vi "GA_Calculate Fitnesses.vi"(6 "Parameters":T1={"Population size"=100, "Generations no."=500, "Significant digits"=4, "Crossover probabality"=0.85, "Mutation mode"=enum."one-point, fixed rate", "Use Gray code?"=FALSE, "Mutation rate"=0.05, "Min mutation rate"=0.0005, "Max mutation rate"=0.25, "Reproduction plan"=enum."Steady-state-replace-worst", "Elitism"=FALSE, "Fmax"=1} {"Max mutation rate" min=0.0 max=1.0; "Min mutation rate" min=0.0 max=1.0; "Mutation rate" min=0.0 max=1.0; "Crossover probabality" min=0.0 max=1.0; "Significant digits" min=1; "Generations no." min=1; "Population size" min=1}, 7 "Fitness Function":T3, 11 "Population in":T2) -> (3 "Population out":T2)   [LabVIEW 2016, in "Optimal Frequency Bands Search.lvlib" / "GeneticAlgorithm.lvlib"]
doc: "Рассчитать значения функции приспособленности"
uses:
  GeneticAlgorithm.lvlib
  GA_tFitness Function.ctl
  GA_tPopulation.ctl
  GA_tParameters.ctl
  particle_swarm_opt/ParticleSwarm.lvlib
panel:
  # "This VI is a part of BCI Design library, http://www.ru-bci.org \nCopyright © 2020, Sotnikov Peter, All rights reserved. License: GNU GPLv3"
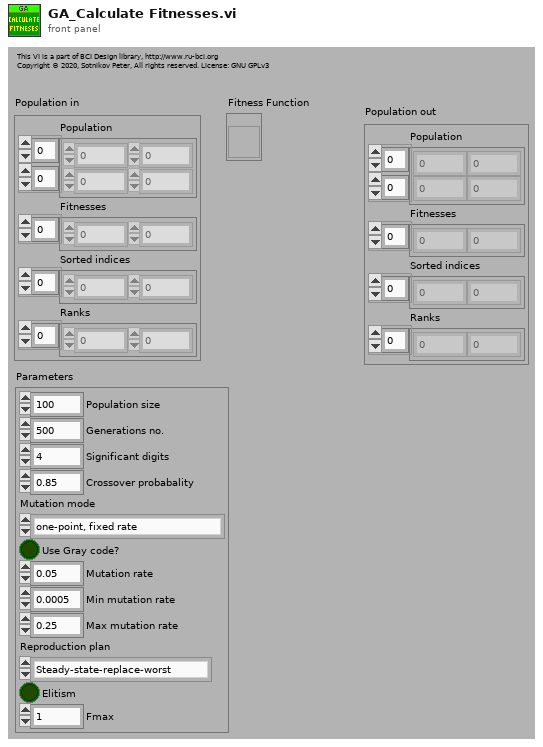
[diagram p1: front panel]
types:
  T1 = typedef "Optimal Frequency Bands Search.lvlib/GeneticAlgorithm.lvlib/GA_tParameters.ctl" = cluster{"Population size":i32, "Generations no.":i32, "Significant digits":i32, "Crossover probabality":dbl, "Mutation mode":enum16{"one-point, fixed rate", "one-point, fitness-adjustable rate", "one-point, distance-adjustable rate"}, "Use Gray code?":bool, "Mutation rate":dbl, "Min mutation rate":dbl, "Max mutation rate":dbl, "Reproduction plan":enum16{"Full generational replacement", "Steady-state-replace-random", "Steady-state-replace-worst"}, "Elitism":bool, "Fmax":i32}
  T2 = typedef "Optimal Frequency Bands Search.lvlib/GeneticAlgorithm.lvlib/GA_tPopulation.ctl" = cluster{"Population":i32[][], "Fitnesses":dbl[], "Sorted indices":i32[], "Ranks":i32[]}
  T3 = typedef "Optimal Frequency Bands Search.lvlib/GeneticAlgorithm.lvlib/GA_tFitness Function.ctl" = refnum<vi>
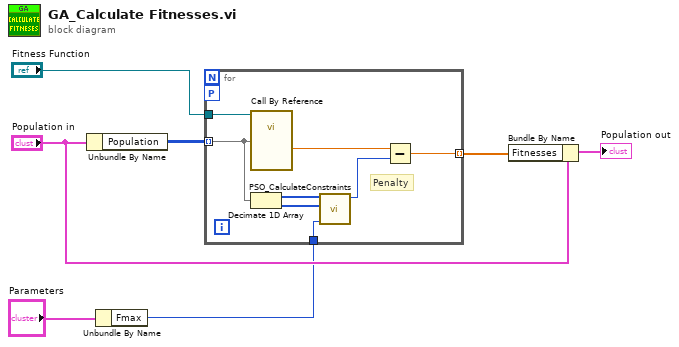
[diagram p0: block diagram]
diagram:
  n1 = Unbundle By Name("Population in") -> ("Population"=w7:i32[][])
  n2 = Unbundle By Name("Parameters") -> ("Fmax"=w1:i32)
  n3 = for {
    tunnel: w7 -> [w13] mode=indexing
    tunnel: "Fitness Function" -> [w15]
    tunnel: [w9] -> w4 mode=indexing
    tunnel: w1 -> [w14]
    workers-P: _ -> [_]
    # "Penalty"
    n4 = call-by-ref "Call By Reference"(reference=w15, "Phenotype"=w13) -> ("Fitness"=w8:dbl)  [unwired: 3 in, 2 out]
    n5 = Decimate 1D Array(w13) -> (w12:i32[], w11:i32[])
    n6 = call "PSO_CalculateConstraints.vi"("Fmax"=w14, "deltaF vector"=w11, "F0 vector"=w12) -> ("Penalty"=w10:i32)  [unwired: 7 in, 1 out]
    n7 = Subtract(x=w8, y=w10) -> (x-y=w9:dbl)
  }
  n8 = Bundle By Name(cluster="Population in", "Fitnesses"=w4) -> (→"Population out":T2)
